vi "Limit Compare.vi"(6 "INFO":T1, 7 "Unit":string, 8 "error in":errorcluster, 9 "Input Data":string, 10 "Limit Signal":string[][](array[string]), 11 "Signal Name":string) -> (0 "error out":errorcluster, 1 "TEST RESULT LOG":T2, 2 "Out range?":bool, 3 "ERROR_LOG":T3, 5 "Log?":bool)   [LabVIEW 2023, in "HardwareAbstractionLayer_LVOOP.lvlib" / "Report.lvclass"]
uses:
  Report.lvclass
  Control/ERROR LOG.ctl
  Control/TEST RESULT LOG.ctl
  Control/FE FF DECODER.ctl
  Report.lvclass/Report.ctl
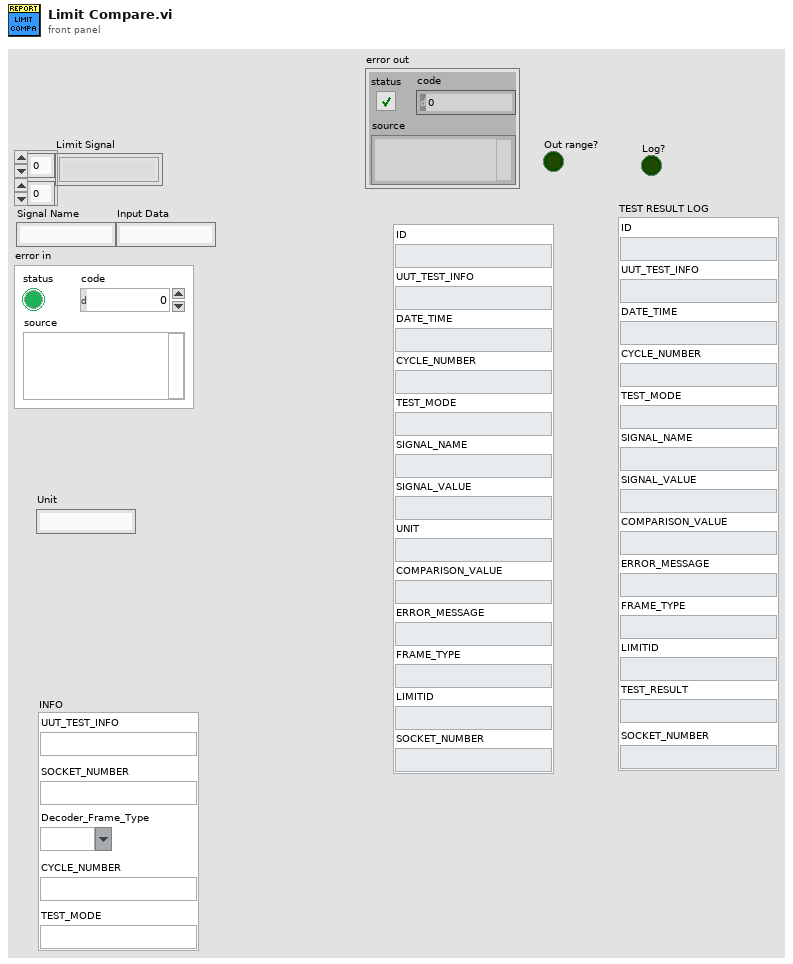
[diagram p1: front panel]
types:
  T1 = typedef "HardwareAbstractionLayer_LVOOP.lvlib/Report.lvclass/FE FF DECODER.ctl" = cluster{"UUT_TEST_INFO":string, "SOCKET_NUMBER":string, "Decoder_Frame_Type":string, "CYCLE_NUMBER":string, "TEST_MODE":string}
  T2 = typedef "HardwareAbstractionLayer_LVOOP.lvlib/Report.lvclass/TEST RESULT LOG.ctl" = cluster{"ID":string, "UUT_TEST_INFO":string, "DATE_TIME":string, "CYCLE_NUMBER":string, "TEST_MODE":string, "SIGNAL_NAME":string, "SIGNAL_VALUE":string, "COMPARISON_VALUE":string, "ERROR_MESSAGE":string, "FRAME_TYPE":string, "LIMITID":string, "TEST_RESULT":string, "SOCKET_NUMBER":string}
  T3 = typedef "HardwareAbstractionLayer_LVOOP.lvlib/Report.lvclass/ERROR LOG.ctl" = cluster{"ID":string, "UUT_TEST_INFO":string, "DATE_TIME":string, "CYCLE_NUMBER":string, "TEST_MODE":string, "SIGNAL_NAME":string, "SIGNAL_VALUE":string, "UNIT":string, "COMPARISON_VALUE":string, "ERROR_MESSAGE":string, "FRAME_TYPE":string, "LIMITID":string, "SOCKET_NUMBER":string}
  T4 = cluster{"Nominal Value":dbl, "Minimum":dbl, "Maximum":dbl, "Tolerance%":dbl}
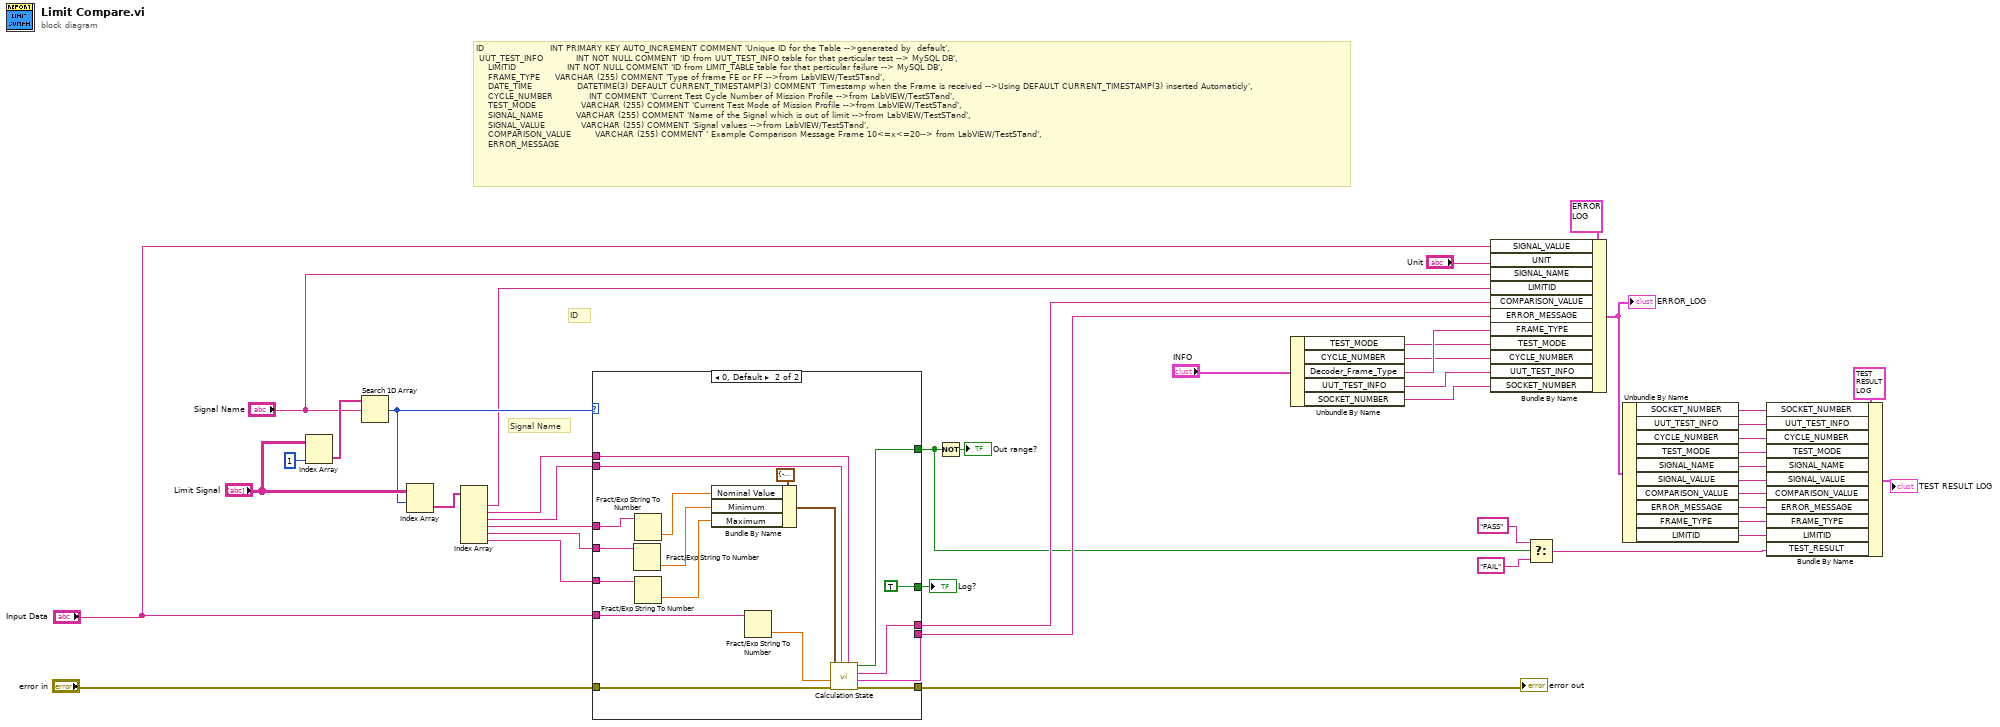
[diagram p0: block diagram]
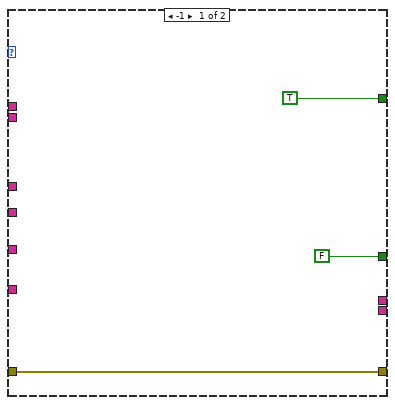
[diagram p2: hidden frame]
diagram:
  # "Signal Name"
  # "ID                      INT PRIMARY KEY AUTO_INCREMENT COMMENT 'Unique ID for the Table -->generated by  default',\n\tUUT_TEST_INFO           INT NOT NULL COMMENT 'ID from UUT_TEST_INFO table for that perticular test --> MySQL DB',\n    LIMITID                 INT NOT NULL COMMENT 'ID from LIMIT_TABLE table for that perticular failure --> MySQL DB',\n    FRAME_TYPE \t\t\t\tVARCHAR (255) COMMENT 'Type of frame FE or FF -->from LabVIEW/TestSTand',\n    DATE_TIME               DATETIME(3) DEFAULT CURRENT_TIMESTAMP(3) COMMENT 'Timestamp when the Frame is received -->Using DEFAULT CURRENT_TIMESTAMP(3) inserted Automaticly',\n    CYCLE_NUMBER            INT COMMENT 'Current Test Cycle Number of Mission Profile -->from LabVIEW/TestSTand',\n    TEST_MODE               VARCHAR (255) COMMENT 'Current Test Mode of Mission Profile -->from LabVIEW/TestSTand',\n    SIGNAL_NAME          \tVARCHAR (255) COMMENT 'Name of the Signal which is out of limit -->from LabVIEW/TestSTand',\n    SIGNAL_VALUE            VARCHAR (255) COMMENT 'Signal values -->from LabVIEW/TestSTand',\n    COMPARISON_VALUE        VARCHAR (255) COMMENT ' Example Comparison Message Frame 10<=x<=20--> from LabVIEW/TestSTand',\n    ERROR_MESSAGE"
  # "ID"
  n1 = Index Array(array="Limit Signal", index (col)=1 ("disabled index (col)")) -> (element=w41:string[])  [unwired: 1 in]
  n2 = Search 1D Array(1D array=w41, element="Signal Name") -> (index of element=w40:i32)  [unwired: 1 in]
  n3 = Index Array(array="Limit Signal", index (row)=w40) -> (element=w39:string[])  [unwired: 1 in]
  n4 = Index Array(array=w39) -> (element #1=w35:string, element #2=w27:string, element #3=w33:string, element #4=w32:string, element #5=w31:string, element #6=w30:string)  [unwired: 6 in]
  n5 = case shown="0, Default" w40 {
    tunnel: "Input Data" -> [_ w65]
    tunnel: [TRUE ("Status") w49] -> w10
    tunnel: "error in" -> [w46 w64]
    tunnel: [w46 w63] -> w44
    tunnel: w32 -> [_ w57]
    tunnel: w31 -> [_ w56]
    tunnel: w30 -> [_ w55]
    tunnel: w33 -> [_ w54]
    tunnel: [_ w53] -> w29
    tunnel: [_ w52] -> w28
    tunnel: w27 -> [_ w51]
    tunnel: [FALSE TRUE] -> w9
    frame -1 {
    }
    frame 0, Default {
      n6 = Fract/Exp String To Number(string=w56) -> (number=w59:dbl)  [unwired: 3 in, 1 out]
      n7 = Fract/Exp String To Number(string=w57) -> (number=w58:dbl)  [unwired: 3 in, 1 out]
      n8 = Fract/Exp String To Number(string=w55) -> (number=w50:dbl)  [unwired: 3 in, 1 out]
      n9 = Bundle By Name(cluster=T4 {"Nominal Value"=-20.0, "Minimum"=-21.0, "Maximum"=-19.0, "Tolerance%"=10.0} ("Signal Limit Data"), "Nominal Value"=w58, "Minimum"=w59, "Maximum"=w50) -> (w60:T4)
      n10 = Fract/Exp String To Number(string=w65) -> (number=w62:dbl)  [unwired: 3 in, 1 out]
      n11 = call "Calculation State.vi"("Signal Name"=w51, "Action"=w54, "error in"=w64, "Signal Values"=w62, "Signal Limit Data"=w60) -> ("error out"=w63:errorcluster, "ERROR MESSAGE"=w52:string, "COMPARISON VALUE"=w53:string, "In Range?"=w49:bool)  [unwired: 3 in]
    }
  }
  "error out" <- w44
  "Log?" <- w9
  n12 = Not(x=w10) -> (.not. x?=→"Out range?":bool)
  n13 = Unbundle By Name("INFO") -> ("TEST_MODE"=w1:string, "CYCLE_NUMBER"=w2:string, "Decoder_Frame_Type"=w4:string, "UUT_TEST_INFO"=w7:string, "SOCKET_NUMBER"=w6:string)
  n14 = Bundle By Name(cluster=T3 {"ID"="", "UUT_TEST_INFO"="", "DATE_TIME"="", "CYCLE_NUMBER"="", "TEST_MODE"="", "SIGNAL_NAME"="", "SIGNAL_VALUE"="", "UNIT"="", "COMPARISON_VALUE"="", "ERROR_MESSAGE"="", "FRAME_TYPE"="", "LIMITID"="", "SOCKET_NUMBER"=""} ("ERROR_LOG"), "SIGNAL_VALUE"="Input Data", "UNIT"="Unit", "SIGNAL_NAME"="Signal Name", "LIMITID"=w35, "COMPARISON_VALUE"=w29, "ERROR_MESSAGE"=w28, "FRAME_TYPE"=w4, "TEST_MODE"=w1, "CYCLE_NUMBER"=w2, "UUT_TEST_INFO"=w7, "SOCKET_NUMBER"=w6) -> (w25:T3)
  "ERROR_LOG" <- w25
  n15 = Select(t="PASS", s=w10, f="FAIL") -> (s? t:f=w14:string)
  n16 = Unbundle By Name(w25) -> ("SOCKET_NUMBER"=w5:string, "UUT_TEST_INFO"=w24:string, "CYCLE_NUMBER"=w16:string, "TEST_MODE"=w17:string, "SIGNAL_NAME"=w18:string, "SIGNAL_VALUE"=w19:string, "COMPARISON_VALUE"=w20:string, "ERROR_MESSAGE"=w21:string, "FRAME_TYPE"=w22:string, "LIMITID"=w23:string)
  n17 = Bundle By Name(cluster=T2 {"ID"="", "UUT_TEST_INFO"="", "DATE_TIME"="", "CYCLE_NUMBER"="", "TEST_MODE"="", "SIGNAL_NAME"="", "SIGNAL_VALUE"="", "COMPARISON_VALUE"="", "ERROR_MESSAGE"="", "FRAME_TYPE"="", "LIMITID"="", "TEST_RESULT"="", "SOCKET_NUMBER"=""} ("ERROR_LOG"), "SOCKET_NUMBER"=w5, "UUT_TEST_INFO"=w24, "CYCLE_NUMBER"=w16, "TEST_MODE"=w17, "SIGNAL_NAME"=w18, "SIGNAL_VALUE"=w19, "COMPARISON_VALUE"=w20, "ERROR_MESSAGE"=w21, "FRAME_TYPE"=w22, "LIMITID"=w23, "TEST_RESULT"=w14) -> (→"TEST RESULT LOG":T2)
